vi "TCP - Open Connection.vi"(8 "error in (no error)":errorcluster, 11 "S7NetCom in":refnum<class "S7NetCom.lvclass">) -> (0 "error out":errorcluster, 3 "S7NetCom out":refnum<class "S7NetCom.lvclass">)   [LabVIEW 2014, in "S7NetCom.lvclass"]
doc: "____\nCopyright (c) 2019 Hampel Software Engineering (HSE), released under BSD license. More info can be found on https://dokuwiki.hampel-soft.com/code/hse/s7netcom. Original code published by Marc Christenson, Sisu Devices."
uses:
  S7NetCom.lvclass
  S7NetCom.lvclass/S7NetCom.ctl
  Accessors/Get IP Address.vi
  Accessors/Get Port.vi
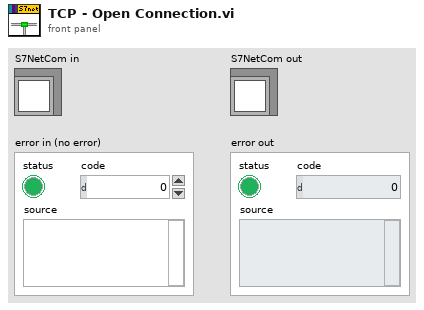
[diagram p1: front panel]
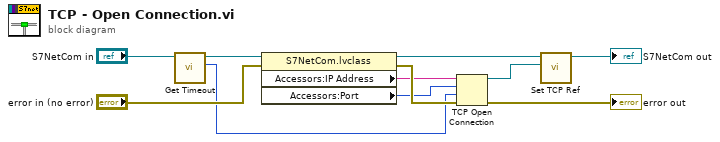
[diagram p0: block diagram]
diagram:
  n1 = call "Get Timeout.vi"("S7NetCom in"="S7NetCom in") -> ("Timeout [ms]"=w3:i32, "S7NetCom out"=w4:refnum<class "S7NetCom.lvclass">)  [unwired: 9 in]
  n2 = property class="S7NetCom.lvclass"(reference=w4, error in="error in (no error)") -> (reference out=w7:refnum<class "S7NetCom.lvclass">, error out=w11:errorcluster, "Accessors:IP Address"=w9:string, "Accessors:Port"=w8:i32)
  n3 = TCP Open Connection(address=w9, remote port or service name=w8, timeout ms (60000)=w3, error in (no error)=w11) -> (connection ID=w1:refnum<k5>, error out=→"error out":errorcluster)  [unwired: 1 out]
  n4 = call "Set TCP Ref.vi"("TCP Ref"=w1, "S7NetCom in"=w7) -> ("S7NetCom out"=→"S7NetCom out":refnum<class "S7NetCom.lvclass">)  [unwired: 9 in]
